vi "Initialization VI.vi"(8 "error in (no error)":errorcluster, 10 "Custom XML":string, 11 "Device Item Ref in":T1 format="%.0x") -> (0 "error out":errorcluster, 3 "Device Item Ref out":T1 format="%.0x")   [LabVIEW 2019, in "Reset Hardware System Explorer.lvlib"]
uses:
  Reset Hardware System Explorer.lvlib
  <vilib>/NI VeriStand/Custom Device API/Custom Device Item Ref.ctl
  <vilib>/NI/NI VeriStand Custom Device Import and Export Tool/ImportExport.lvlib
  <vilib>/NI VeriStand/Custom Device API/Custom Device API.lvlib
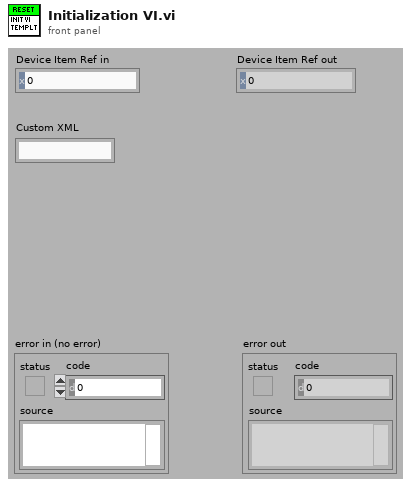
[diagram p1: front panel]
types:
  T1 = typedef "Custom Device API.lvlib/Custom Device Item Ref.ctl" = u64
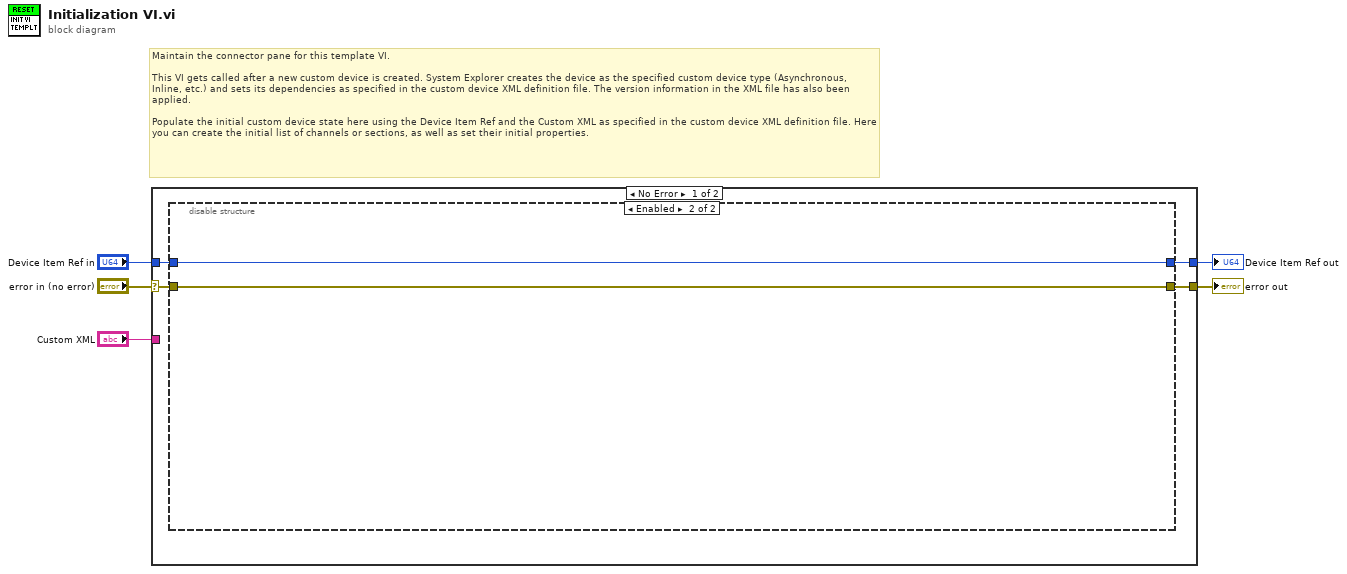
[diagram p0: block diagram]
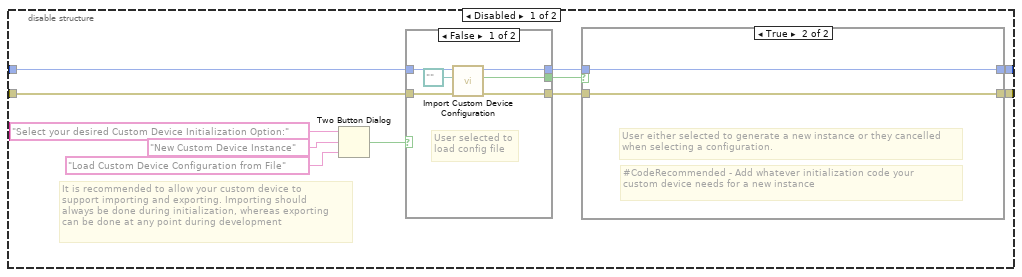
[diagram p2: hidden frame]
diagram:
  # "Maintain the connector pane for this template VI.\n\nThis VI gets called after a new custom device is created. System Explorer creates the device as the specified custom device type (Asynchronous, Inline, etc.) and sets its dependencies as specified in the custom device XML definition file. The version information in the XML file has also been applied.\n\nPopulate the initial custom device state here using the Device Item Ref and the Custom XML as specified in the custom device XML definition file. Here you can create the initial list of channels or sections, as well as set their initial properties."
  n1 = case shown="No Error" "error in (no error)" {
    selector: "error in (no error)" -> [w8 w37]
    tunnel: [w7 w37] -> w5
    tunnel: [w6 w36] -> w3
    tunnel: "Device Item Ref in" -> [w9 w36]
    tunnel: "Custom XML" -> [_ _]
    frame No Error {
      n2 = disable-structure shown="Enabled" {
        disable-tunnel: w9 -> [w16 w35]
        disable-tunnel: w8 -> [w15 w34]
        disable-tunnel: [w11 w34] -> w7
        disable-tunnel: [w10 w35] -> w6
        frame Disabled {
          # "It is recommended to allow your custom device to\nsupport importing and exporting. Importing should\nalways be done during initialization, whereas exporting\ncan be done at any point during development"
          n3 = Two Button Dialog(message="Select your desired Custom Device Initialization Option:", 1:"Load Custom Device Configuration from File" ("F button name (\"Cancel\")"), 2:"New Custom Device Instance" ("T button name (\"OK\")")) -> (T button?=w17:bool)
          n4 = case shown="False" w17 {
            selector: w17 -> [_ w31]
            tunnel: w16 -> [w30 w33]
            tunnel: [w29 w33] -> w14
            tunnel: w15 -> [w27 w32]
            tunnel: [w26 w32] -> w12
            tunnel: [w25 w31] -> w13
            frame False {
              # "User selected to\nload config file"
              n5 = call <vilib>:"Import Custom Device Configuration.vi"("error in (no error)"=w27, "Path"=path "", "NodeID"=w30) -> ("error out"=w26:errorcluster, "cancelled"=w25:bool, "NodeID out"=w29:u64)  [unwired: 6 in]
            }
            frame True {
              # "User selected new\ncustom device. Do\nnothing in this case\nand handle new\ngeneration in the\nnext case structure"
            }
          }
          n6 = case shown="True" w13 {
            tunnel: w14 -> [w22 w23]
            tunnel: w12 -> [w21 w24]
            tunnel: [w21 w24] -> w11
            tunnel: [w22 w23] -> w10
            frame False {
              # "User selected to import from configuration and didn't cancel import"
            }
            frame True {
              # "#CodeRecommended - Add whatever initialization code your\ncustom device needs for a new instance"
              # "User either selected to generate a new instance or they cancelled\nwhen selecting a configuration."
            }
          }
        }
        frame Enabled {
        }
      }
    }
    frame Error {
    }
  }
  "error out" <- w5
  "Device Item Ref out" <- w3
